vi "ContourFilledAuto0008.vi"   [LabVIEW 2013]
uses:
  <vilib>/Heliosphere Research LLC/Advanced Plotting Toolkit/api_core/NewPlotScales.ctl
  ErrorCodes.ctl
  <vilib>/Heliosphere Research LLC/Advanced Plotting Toolkit/api_plotting/ContourFilled_Automatic.vi
  <vilib>/Heliosphere Research LLC/Advanced Plotting Toolkit/Advanced Plotting Toolkit.lvlib
types:
  T1 = typedef "ErrorCodes.ctl" = u32
  T2 = typedef "Advanced Plotting Toolkit.lvlib/NewPlotScales.ctl" = enum16{"Default", "Linear", "Log", "Symlog"}
  T3 = typedef "Advanced Plotting Toolkit.lvlib/PlotID.ctl" = i32
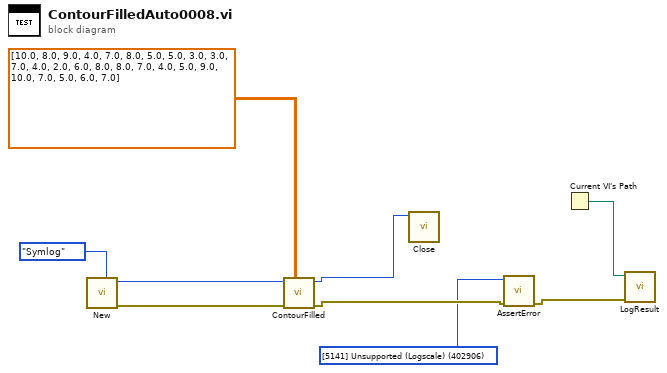
[diagram p0: block diagram]
diagram:
  w1 = T1 402906 items=["[5120] Invalid ID"=402902, "[5110] Failed to Init"=402900, "[5111] Unknown Error"=402901, "[5130] Save - Bad File Extension"=402403, "[5131] Save - General Error"=402904, "[5140] Unsupported (Polar)"=402905, "[5141] Unsupported (Logscale)"=402906, "[5142] Coordinates Not Regular"=402907] ("Expected Error")
  n1 = call <vilib>:"New.vi"("Y Axis Scale"=NewPlotScales."Symlog") -> ("error out"=w5:errorcluster, "Plot ID"=w6:T3)  [unwired: 9 in]
  n2 = call-poly <vilib>:"ContourFilled.vi"("Z Data"=dbl[][] [[10.0, 8.0, 9.0, 4.0, 7.0], [8.0, 5.0, 5.0, 3.0, 3.0], [7.0, 4.0, 2.0, 6.0, 8.0], [8.0, 7.0, 4.0, 5.0, 9.0], [10.0, 7.0, 5.0, 6.0, 7.0]], "error in (no error)"=w5, "Plot ID"=w6) -> ("error out"=w4:errorcluster, "Plot ID Out"=w3:T3)  [unwired: 7 in]
  n3 = call <vilib>:"Close.vi"("Plot ID"=w3) -> ()  [unwired: 10 in, 1 out]
  n4 = call "AssertError.vi"("error in (no error)"=w4, "Expected Error"=w1) -> ("error out"=w2:errorcluster)  [unwired: 9 in]
  n5 = Current VI's Path() -> (path=w9:path)
  n6 = call "LogResult.vi"("Test Result"=w2, "VI Path"=w9) -> ()  [unwired: 10 in]
